vi "DecodeMonitorHeader(FHTW).vi"(11 "fhtw":u32 format="%.0x") -> (3 "header type":u32)   [LabVIEW 2020, in "AIM664LV.lvlib"]
uses:
  AIM664LV.lvlib
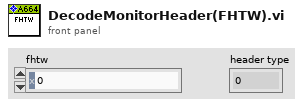
[diagram p1: front panel]
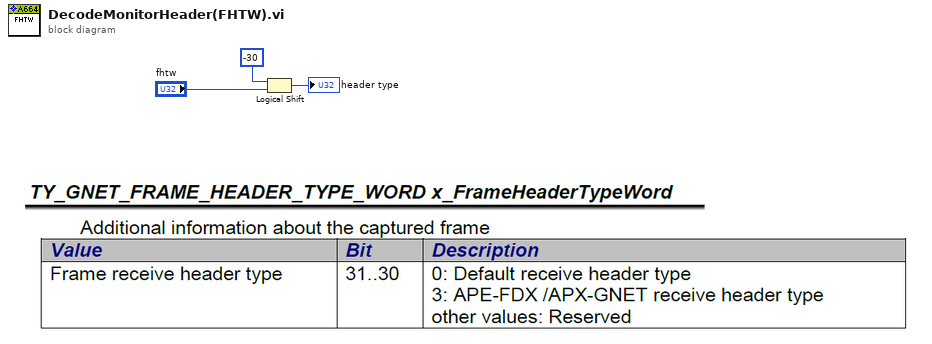
[diagram p0: block diagram]
diagram:
  n1 = Logical Shift(y=i16 -30, x="fhtw") -> (x << y=→"header type":u32)
